vi "ChangeBaseSavePath.vi"() -> (3 "selected path":path)   [LabVIEW 2014]
uses:
  <vilib>/Utility/config.llb/Write Key (String).vi
  <vilib>/Utility/config.llb/NI_LVConfig.lvlib
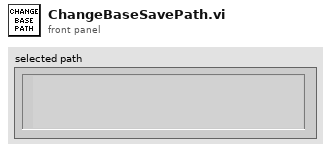
[diagram p1: front panel]
types:
  T1 = typedef "NI_LVConfig.lvlib/Config Data RefNum.ctl" = refnum<k1>
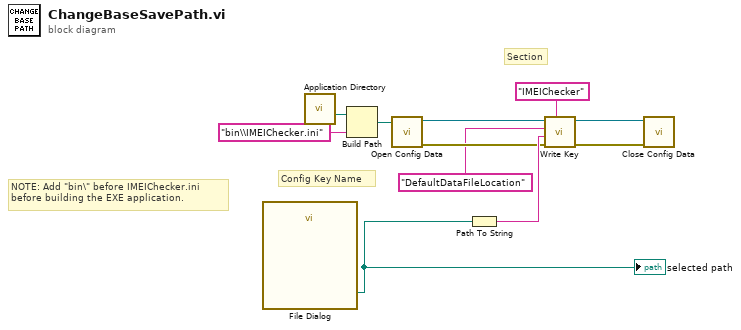
[diagram p0: block diagram]
diagram:
  # "NOTE: Add \"bin\\\" before IMEIChecker.ini\nbefore building the EXE application."
  # "Config Key Name"
  # "Section"
  n1 = call "File Dialog"() -> ("selected path"=w1:path)  [unwired: 12 in, 3 out]
  "selected path" <- w1
  n2 = call <vilib>:"Application Directory.vi"() -> ("Application Directory"=w9:path)
  n3 = Build Path(base path=w9, name or relative path="bin\\IMEIChecker.ini") -> (appended path=w11:path)
  n4 = call <vilib>:"Open Config Data.vi"("configuration file path"=w11) -> ("error out"=w5:errorcluster, "refnum"=w4:T1)  [unwired: 8 in, 1 out]
  n5 = Path To String(path=w1) -> (string=w8:string)
  n6 = call-poly <vilib>:"Write Key.vi"("section"="IMEIChecker", "error in (no error)"=w5, "value"=w8, "key"="DefaultDataFileLocation", "refnum"=w4) -> ("error out"=w7:errorcluster, "refnum out"=w6:T1)  [unwired: 4 in, 1 out]
  n7 = call <vilib>:"Close Config Data.vi"("error in (no error)"=w7, "refnum"=w6) -> ()  [unwired: 8 in, 2 out]
